vi "SetWindowShape.vi"(8 "No Error":errorcluster, 10 "Shape [SDL_Surface *] (0: Remove Current)":i64 format="%.0x", 11 "Window [SDL_Window *]":i64 format="%.0x") -> (0 "Error Out":errorcluster)   [LabVIEW 2026, in "SDL3.lvlib" / "Video.lvlib"]
doc: "<B>Summary</B>\nSet the shape of a transparent window.\n\n<B>Remarks</B>\nThis sets the alpha channel of a transparent window and any fully transparent areas are also transparent to mouse clicks. If you are using something besides the SDL render API, then you are responsible for drawing the alpha channel of the window to match the shape alpha channel to get consistent cross-platform results.\n\nThe shape is copied inside this function, so you can free it afterwards. If your shape surface changes, you should call <B>SDL_SetWindowShape()</B> again to update the window. This is an expensive operation, so should be done sparingly.\n\nThe window must have been created with the <B>SDL_WINDOW_TRANSPARENT</B> flag."
uses:
  Video.lvlib
  <vilib>/Utility/error.llb/Error Cluster From Error Code.vi
  Error/Error.lvlib
  Lib/SDL3.dll
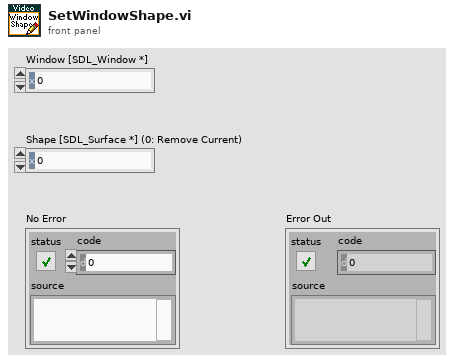
[diagram p1: front panel]
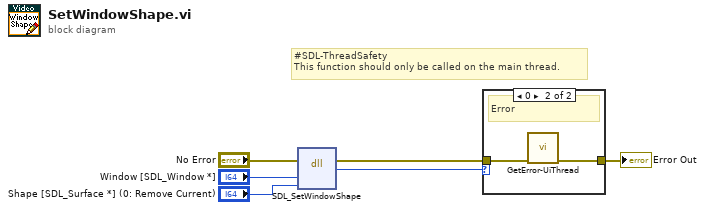
[diagram p0: block diagram]
diagram:
  # "#SDL-ThreadSafety\nThis function should only be called on the main thread."
  n1 = dll-call lib="C:/Users/saukko/Dev/LV-SDL3/Sources/SDL3/Lib/SDL3.*" fn="SDL_SetWindowShape"(error in="No Error", "window"="Window [SDL_Window *]", "shape"="Shape [SDL_Surface *] (0: Remove Current)") -> (error out=w3:errorcluster, "return type"=w2:i32)  [unwired: 4 in, 1 out]
  n2 = case shown="0" w2 {
    tunnel: w3 -> [w7 w9]
    tunnel: [w7 w8] -> w5
    frame Default {
      # "Ok"
    }
    frame 0 {
      # "Error"
      n3 = call "GetError-UiThread.vi"("No Error"=w9) -> ("error out"=w8:errorcluster)  [unwired: 10 in]
    }
  }
  "Error Out" <- w5
